vi "navX GetRefnum.vi"(8 "error in (no error)":errorcluster, 10 "refnum name":string) -> (0 "error out":errorcluster, 3 "navX Device TypeDef":T1={"navX Interface Protocol"=enum."SPI", "navX Interface Protocol TypeDefs"={"SPIDevRef"={"DevStatus"={"status"=FALSE, "code"=0, "source"=""}, "Handle"=0, "Controller"=enum."Controller 1", "SPI Bus"=enum."SPI On-Board, CS0"}, "I2CDevRef"={"DevStatus"={"status"=FALSE, "code"=0, "source"=""}, "Controller"=enum."Controller 1", "Device Address"=0, "Handle"=0, "I2C Bus"=enum."Invalid"}, "SerialPortRef"={"DevStatus"={"status"=FALSE, "code"=0, "source"=""}, "Serial Port Name"=""}}, "navX System Information"={"Board Information"={"WhoAmI (50 | 0x32)"=0, "Board Revision"=0, "Firmware Major Version"=0, "Firmware Minor Version"=0, "NAVX_BOARD_CAPABILITY"={"OMNIMOUNT"=FALSE, "YAW_RESET"=FALSE, "VEL_AND_DISP"=FALSE}, "NAVX_BOARD_YAW_AXIS"={"BOARD_YAW_AXIS_UP"=FALSE, "BOARD_YAW_AXIS"=0}}, "Status"={"Update Rate Hz"=0, "Accelerometer Full-Scale Range"=0, "Gyro Full-Scale Range"=0, "NAVX_OP_STATUS"=0, "NAVX_CAL_STATUS"=0, "NAVX_SELFTEST_STATUS"=0, "NAVX_SENSOR_STATUS"={"MOVING"=FALSE, "YAW_STABLE"=FALSE, "MAG_DISTURBANCE"=FALSE, "ALTITUDE_VALID"=FALSE, "SEALEVEL_PRESS_SET"=FALSE, "FUSED_HEADING_VALID"=FALSE}}, "Offsets"={"Yaw"=0.0, "Quat W"=0.0, "Quat X"=0.0, "Quat Y"=0.0, "Quat Z"=0.0}, "LastSampleTimestamp"=0.0, "LastSampleValid"=FALSE}, "navX Common Information"={"Update Rate (4Hz-60Hz)"=50, "refnum name"="", "error"={"status"=FALSE, "code"=0, "source"=""}, "LastFPGATimestamp"=0.0, "Reboot Detected"=FALSE}, "Serial Protocol Extra"={"Loop VI Refnum"=refnum, "Nav6Mode (YPR)"=enum."Raw"}} {"navX Common Information"."Update Rate (4Hz-60Hz)" min=4 max=60 step=1; "navX System Information"."Status"."NAVX_OP_STATUS" items=["INITIALIZING", "SELFTEST_IN_PROGRESS", "ERROR", "IMU_AUTOCAL_IN_PROGRESS", "NORMAL"]; "navX System Information"."Status"."NAVX_CAL_STATUS" items=["IMU_CAL_STATE_MASK"=3, "IMU_CAL_INPROGRESS"=0, "IMU_CAL_ACCUMULATE"=1, "IMU_CAL_COMPLETE"=2, "MAG_CAL_COMPLETE"=4, "BARO_CAL_COMPLETE"=8]; "navX System Information"."Status"."NAVX_SELFTEST_STATUS" items=["COMPLETE"=80, "GYRO_PASSED"=1, "ACCEL_PASSED"=2, "MAG_PASSED"=4, "BARO_PASSED"=8]; "navX Interface Protocol TypeDefs"."I2CDevRef"."Device Address" format="%.0x"})   [LabVIEW 2014, in "navX Library v1 (deprecated).lvlib"]
doc: "This VI gets the refnum for a navX MXP unit."
uses:
  navX Library v1 (deprecated).lvlib
  TypeDefs/navX Device TypeDef.ctl
  TypeDefs/Value TypeDefs/navX Interface Protocol.ctl
  <vilib>/Rock Robotics/WPI/SPI/WPI_SPIDevRef.ctl
  <vilib>/Rock Robotics/SystemInterfaces/Typedef/FPGA_TypedefDigitalModule.ctl
  <vilib>/Rock Robotics/SystemInterfaces/spilib/spi_bus.ctl
  <vilib>/Rock Robotics/WPI/I2C/WPI_I2CDevRef.ctl
  <vilib>/Rock Robotics/SystemInterfaces/i2clib/i2c_bus.ctl
  <vilib>/Rock Robotics/WPI/SerialPort/WPI_SerialPortRef.ctl
  TypeDefs/Data TypeDefs/navX Board Information.ctl
  TypeDefs/Value TypeDefs/navX NAVX_BOARD_CAPABILITY.ctl
  TypeDefs/Value TypeDefs/navX NAVX_BOARD_YAW_AXIS.ctl
  TypeDefs/Data TypeDefs/navX Status Data.ctl
  TypeDefs/Value TypeDefs/navX NAVX_OP_STATUS.ctl
  TypeDefs/Value TypeDefs/navX NAVX_CAL_STATUS.ctl
  TypeDefs/Value TypeDefs/navX NAVX_SELFTEST_STATUS.ctl
  TypeDefs/Value TypeDefs/navX NAVX_SENSOR_STATUS.ctl
  TypeDefs/Data TypeDefs/navX Offsets Data.ctl
  TypeDefs/Value TypeDefs/navX Update Rate.ctl
  TypeDefs/Value TypeDefs/navX Serial Mode.ctl
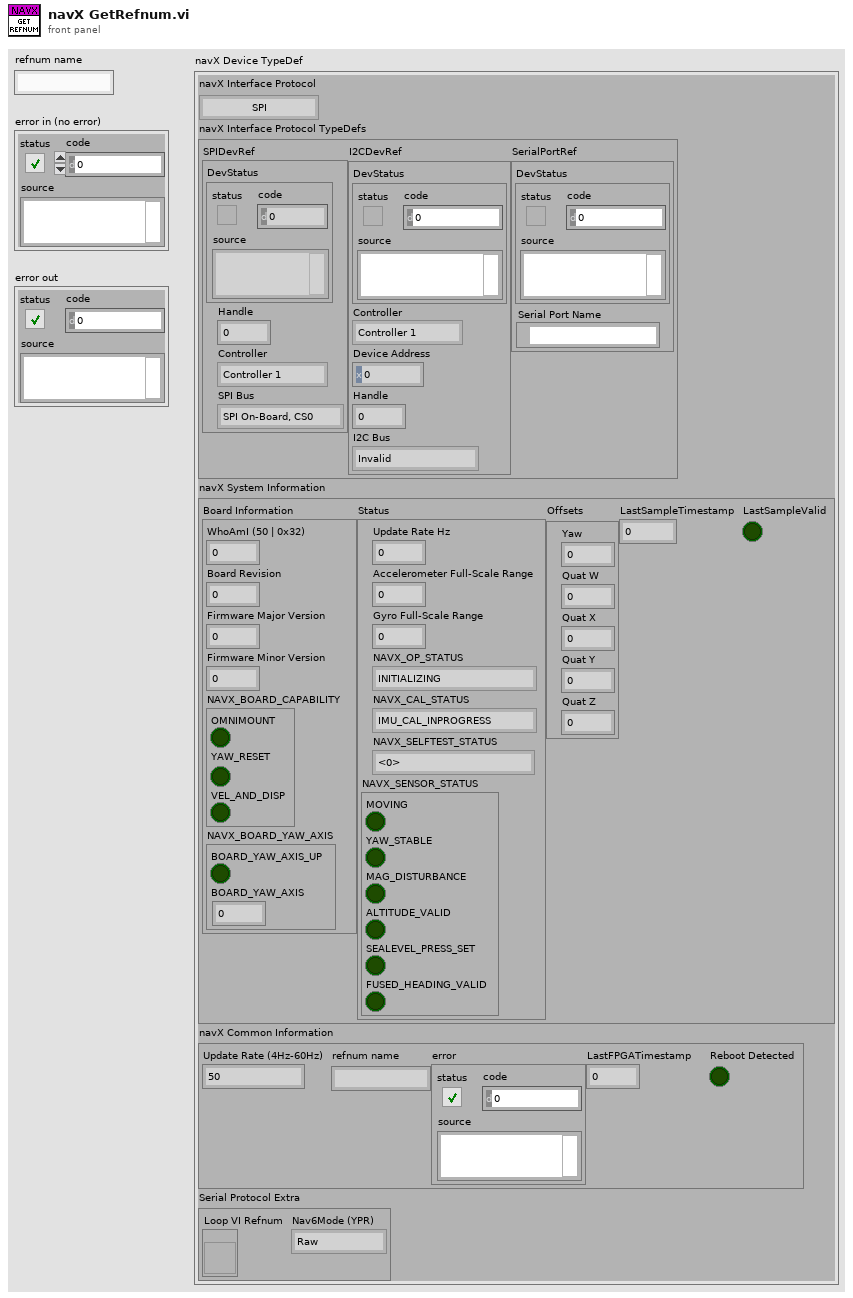
[diagram p1: front panel]
types:
  T1 = typedef "navX Library v1 (deprecated).lvlib/navX Device TypeDef.ctl" = cluster{"navX Interface Protocol":T2, "navX Interface Protocol TypeDefs":cluster{"SPIDevRef":T3, "I2CDevRef":T6, "SerialPortRef":T8}, "navX System Information":cluster{"Board Information":T9, "Status":T12, "Offsets":T17, "LastSampleTimestamp":dbl, "LastSampleValid":bool}, "navX Common Information":cluster{"Update Rate (4Hz-60Hz)":T18, "refnum name":string, "error":errorcluster, "LastFPGATimestamp":dbl, "Reboot Detected":bool}, "Serial Protocol Extra":cluster{"Loop VI Refnum":refnum<vi>, "Nav6Mode (YPR)":T19}}
  T2 = typedef "navX Library v1 (deprecated).lvlib/navX Interface Protocol.ctl" = enum16{"SPI", "I2C", "SERIAL"}
  T3 = typedef "WPI_SPIDevRef.ctl" = cluster{"DevStatus":errorcluster, "Handle":i32, "Controller":T4, "SPI Bus":T5}
  T4 = typedef "FPGA_TypedefDigitalModule.ctl" = enum16{"Controller 1"}
  T5 = typedef "spi_bus.ctl" = enum16{"SPI On-Board, CS0", "SPI On-Board, CS1", "SPI On-Board, CS2", "SPI On-Board, CS3", "SPI MXP", "Invalid"}
  T6 = typedef "WPI_I2CDevRef.ctl" = cluster{"DevStatus":errorcluster, "Controller":T4, "Device Address":u8, "Handle":i32, "I2C Bus":T7}
  T7 = typedef "i2c_bus.ctl" = enum16{"I2C On-Board", "I2C MXP", "Invalid"}
  T8 = typedef "WPI_SerialPortRef.ctl" = cluster{"DevStatus":errorcluster, "Serial Port Name":refnum<visa-resource-name>}
  T9 = typedef "navX Library v1 (deprecated).lvlib/navX Board Information.ctl" = cluster{"WhoAmI (50 | 0x32)":u8, "Board Revision":u8, "Firmware Major Version":u8, "Firmware Minor Version":u8, "NAVX_BOARD_CAPABILITY":T10, "NAVX_BOARD_YAW_AXIS":T11}
  T10 = typedef "navX Library v1 (deprecated).lvlib/navX NAVX_BOARD_CAPABILITY.ctl" = cluster{"OMNIMOUNT":bool, "YAW_RESET":bool, "VEL_AND_DISP":bool}
  T11 = typedef "navX Library v1 (deprecated).lvlib/navX NAVX_BOARD_YAW_AXIS.ctl" = cluster{"BOARD_YAW_AXIS_UP":bool, "BOARD_YAW_AXIS":u8}
  T12 = typedef "navX Library v1 (deprecated).lvlib/navX Status Data.ctl" = cluster{"Update Rate Hz":u8, "Accelerometer Full-Scale Range":u8, "Gyro Full-Scale Range":u16, "NAVX_OP_STATUS":T13, "NAVX_CAL_STATUS":T14, "NAVX_SELFTEST_STATUS":T15, "NAVX_SENSOR_STATUS":T16}
  T13 = typedef "navX Library v1 (deprecated).lvlib/navX NAVX_OP_STATUS.ctl" = u8
  T14 = typedef "navX Library v1 (deprecated).lvlib/navX NAVX_CAL_STATUS.ctl" = u8
  T15 = typedef "navX Library v1 (deprecated).lvlib/navX NAVX_SELFTEST_STATUS.ctl" = u8
  T16 = typedef "navX Library v1 (deprecated).lvlib/navX NAVX_SENSOR_STATUS.ctl" = cluster{"MOVING":bool, "YAW_STABLE":bool, "MAG_DISTURBANCE":bool, "ALTITUDE_VALID":bool, "SEALEVEL_PRESS_SET":bool, "FUSED_HEADING_VALID":bool}
  T17 = typedef "navX Library v1 (deprecated).lvlib/navX Offsets Data.ctl" = cluster{"Yaw":dbl, "Quat W":dbl, "Quat X":dbl, "Quat Y":dbl, "Quat Z":dbl}
  T18 = typedef "navX Library v1 (deprecated).lvlib/navX Update Rate.ctl" = u8
  T19 = typedef "navX Library v1 (deprecated).lvlib/navX Serial Mode.ctl" = enum16{"Raw", "Processed"}
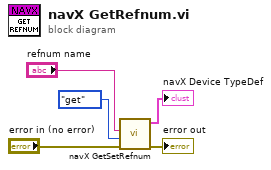
[diagram p0: block diagram]
diagram:
  n1 = call "navX GetSetRefnum.vi"("error in (no error)"="error in (no error)", "Access Type"=enum16{"set", "get", "delete"}."get" ("menu"), "refnum name"="refnum name") -> ("error out"=→"error out":errorcluster, "navX Device TypeDef"=→"navX Device TypeDef":T1)  [unwired: 7 in]
